vi "Host_HoppingScan(XZ_TargetMultiLayerImage).vi"() -> ()   [LabVIEW 2014]
uses:
  <vilib>/userdefined/High Color/nirio_resource_hc.ctl
  <vilib>/Instr/_visa.llb/VISA Configure Serial Port (Instr).vi
  <vilib>/FPGAPlugInAG/PCIe-7851R/niLvFpga_Open_PCIe-7851R.vi
  <vilib>/rvi/interface/common/dynamic/niFpgaDynamicAddResources.vi
  <vilib>/Utility/error.llb/Error Cluster From Error Code.vi
  <vilib>/rvi/errors/niLvFpgaAdjustHostInterfaceError.vi
  <vilib>/FPGAPlugInAG/Dynamic/niLvFpga_Close_Dynamic.vi
  <vilib>/rvi/interface/nirviOpenFPGA/nirviOpenFPGA.xnode
  FPGA Bitfiles/XZFPGAWithinHopp_FPGATarget_HoppingStep(Nonl_hC1Fmxzhga8.lvbitx
  <vilib>/rvi/interface/nirviReadWriteControl/nirviReadWriteControl.xnode
  <vilib>/rvi/interface/nirviMethod/nirviMethod.xnode
  <vilib>/rvi/interface/nirviCloseFPGA/nirviCloseFPGA.xnode
  NiFpgaLv.dll
  <vilib>/rvi/interface/Simulation/niFpgaSimulationCallBeginRW.vi
  <vilib>/FPGAPlugInAG/Dynamic/niLvFpga_ReadFifo_Dynamic.vi
  <vilib>/rvi/errors/niLvFpgaMergeErrorWithErrorCode.vi
  <vilib>/FPGAPlugInAG/Dynamic/niLvFpga_StopFifo_Dynamic.vi
panel:
  out "RTPlot":i32(graph)
  in  "ScanLayerNum":u32
  in  "LowPassFilter":i32
  out "XGetNum":u32
  in  "BottomSleep us":i32
  in  "UpperSleep us":i32
  out "SecElapsed s":dbl
  in  "UseCompensation":bool
  in  "Compensation / line":i32
  in  "RelativeWithdraw index":i32
  out "YPresPos":i32
  out "XBuffer":u32
  out "LinePlot":i16[](graph)
  in  "stop":bool
  in  "ZOffset index":i32
  out "YPos?":dbl
  in  "YNum":i16
  in  "XNum":i16
  in  "YStepLen um":dbl format="%#_13g"
  in  "XStepMultiplier / 0.5nm":i16
  in  "XInitPos um":dbl format="%#_13g"
  in  "YInitPos um":dbl format="%#_13g"
  in  "PIXZ":T1
  out "ERR?":string
  in  "PIYDigital":refnum<visa-resource-name>
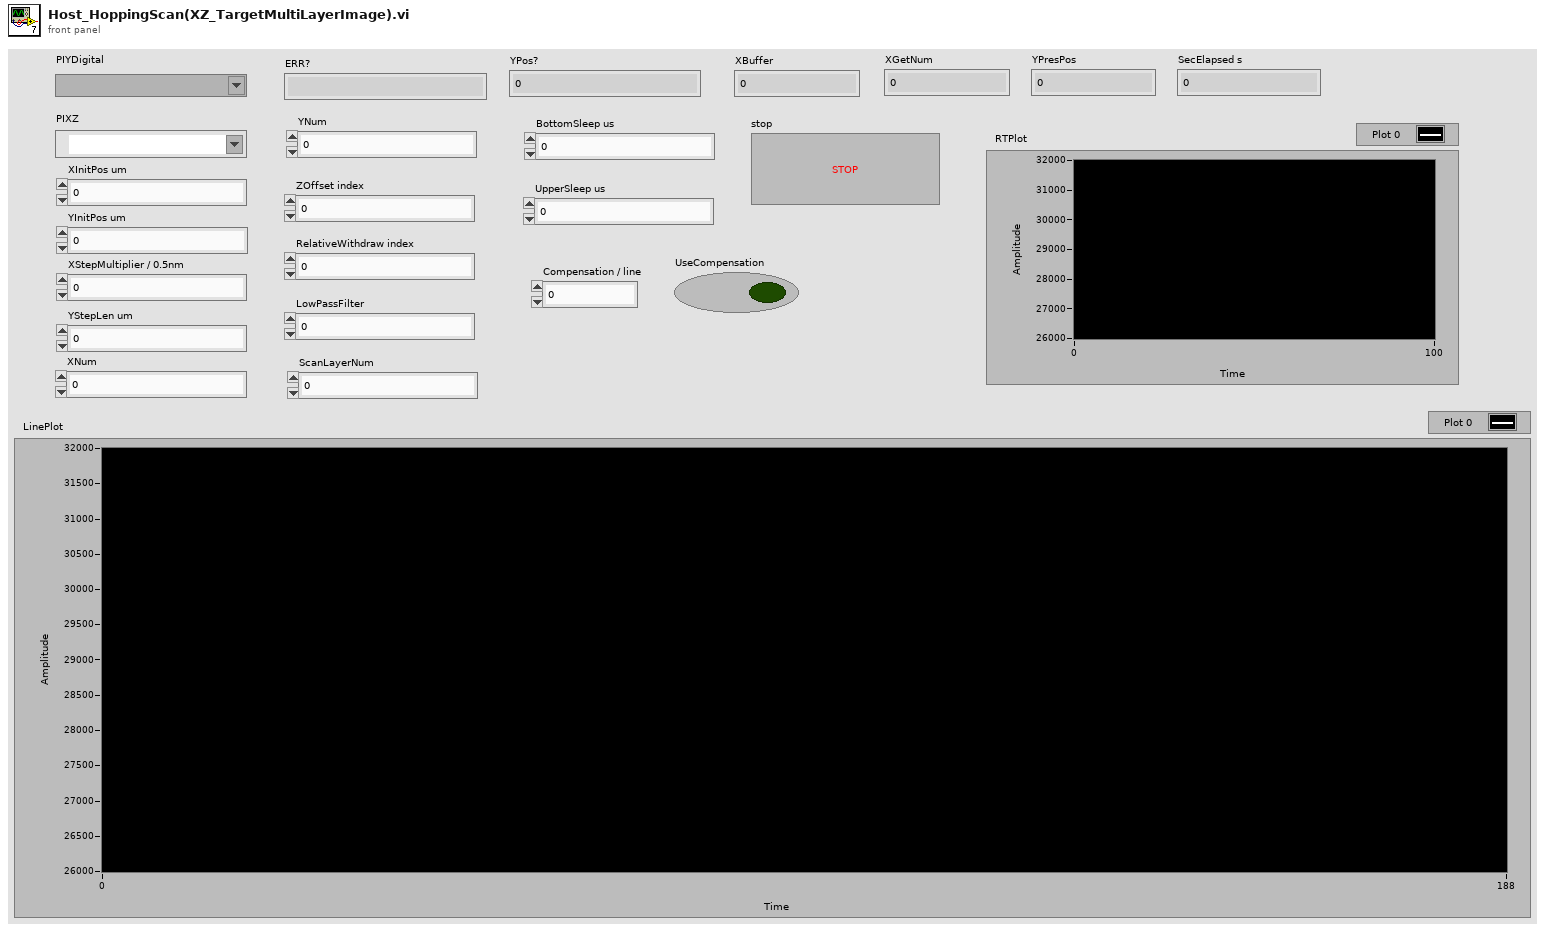
[diagram p1: front panel]
types:
  T1 = typedef "nirio_resource_hc.ctl" = tag
  T2 = enum16{"open", "replace", "create", "open or create", "replace or create", "replace or create with confirmation"}
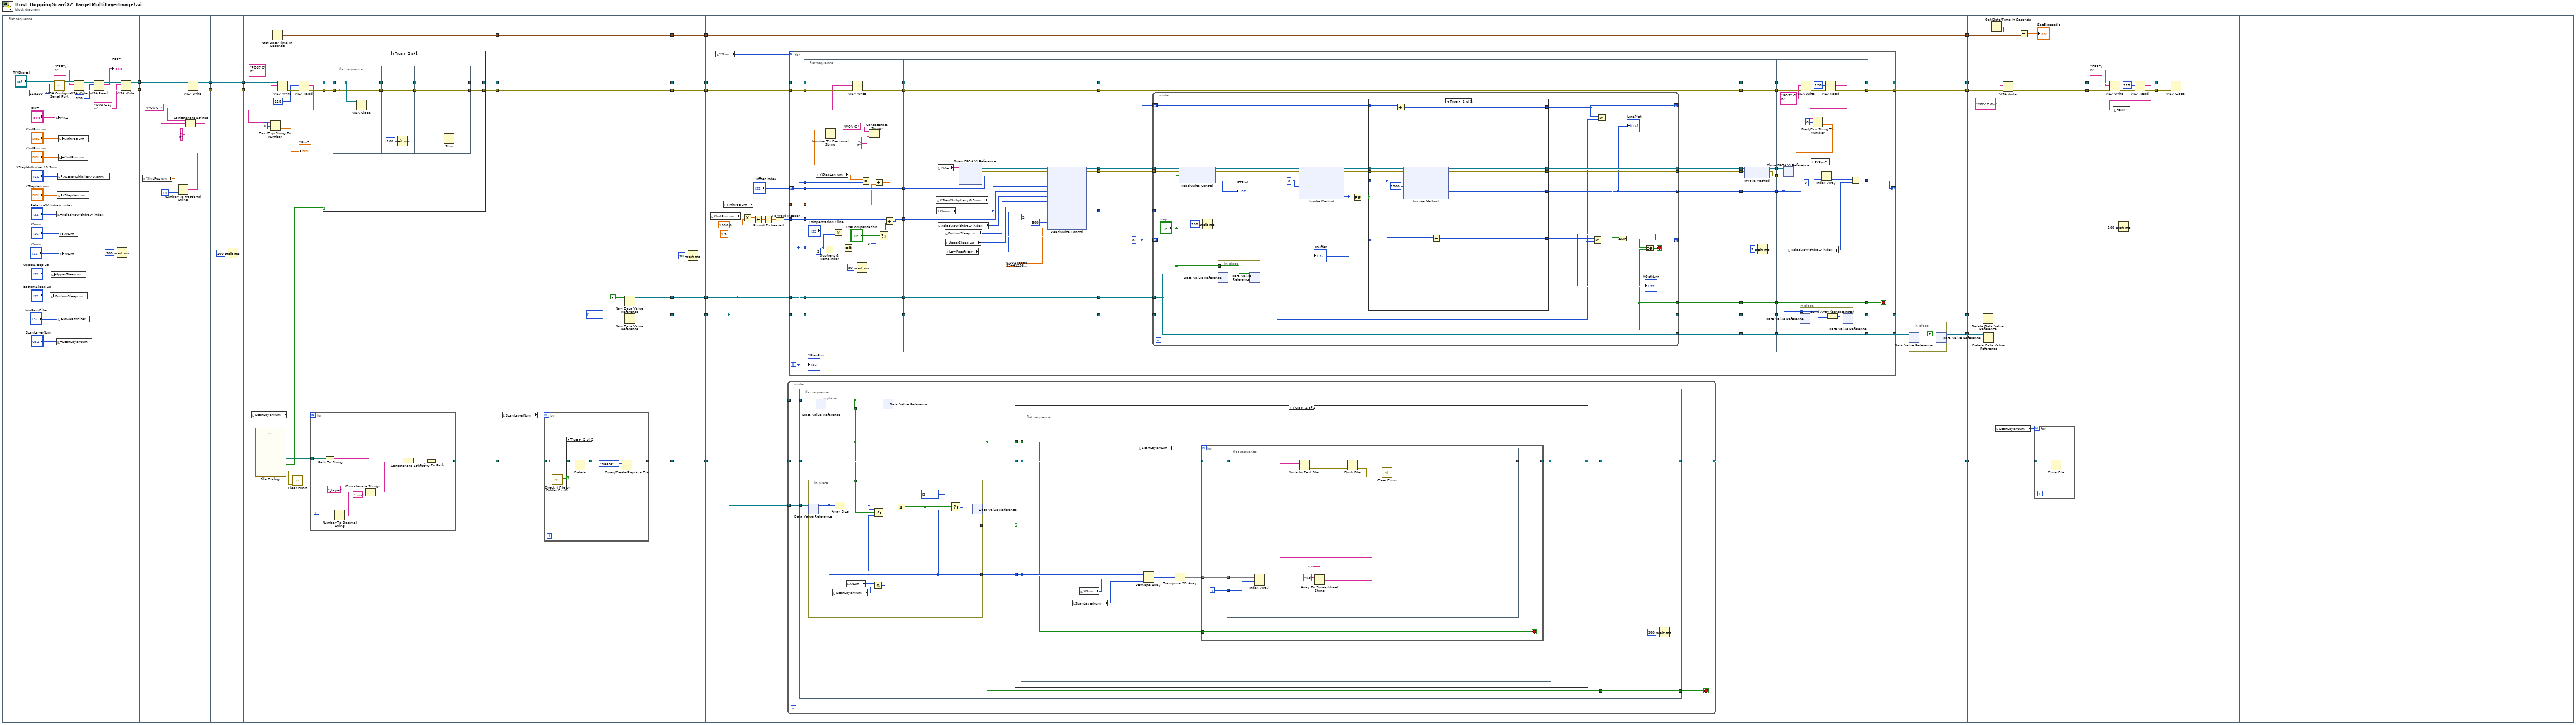
[diagram p0: block diagram]
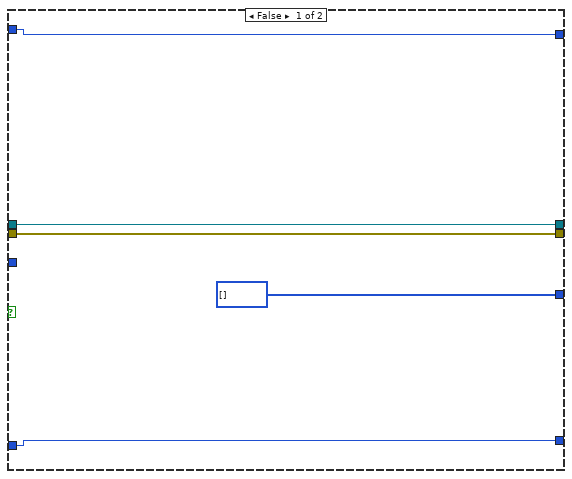
[diagram p5: hidden frame]
diagram:
  n1 = flat-sequence {
    tunnel: [w39] -> w32
    tunnel: [w38] -> w31
    tunnel: w32 -> [w69]
    tunnel: w31 -> [w68]
    tunnel: [w64] -> w30
    tunnel: [w63] -> w29
    tunnel: w30 -> [w71]
    tunnel: w29 -> [w70]
    tunnel: [w71] -> w28
    tunnel: [w70] -> w27
    tunnel: w28 -> [w91]
    tunnel: w27 -> [w90]
    tunnel: [w78] -> w16
    tunnel: [w77] -> w14
    tunnel: [w82] -> w12
    tunnel: [w73] -> w10
    tunnel: w16 -> [w127]
    tunnel: [w127] -> w15
    tunnel: w14 -> [w126]
    tunnel: [w126] -> w13
    tunnel: w12 -> [w125]
    tunnel: [w125] -> w11
    tunnel: w10 -> [w123]
    tunnel: [w122] -> w8
    tunnel: [w120] -> w6
    tunnel: [w118] -> w4
    tunnel: w15 -> [w141]
    tunnel: w13 -> [w140]
    tunnel: [w141] -> w26
    tunnel: [w140] -> w25
    tunnel: [w139] -> w18
    tunnel: w11 -> [w139]
    tunnel: [w138] -> w9
    tunnel: w8 -> [w138]
    tunnel: [w137] -> w7
    tunnel: w6 -> [w137]
    tunnel: [w136] -> w5
    tunnel: w4 -> [w136]
    tunnel: w26 -> [w163]
    tunnel: w25 -> [w162]
    tunnel: [w154] -> w24
    tunnel: [w153] -> w23
    tunnel: w18 -> [w150]
    tunnel: [w150] -> w17
    tunnel: w9 -> [w149]
    tunnel: w7 -> [w148]
    tunnel: w5 -> [w147]
    tunnel: [w145] -> w3
    tunnel: [w144] -> w2
    tunnel: [w143] -> w1
    tunnel: w24 -> [w418]
    tunnel: w23 -> [w417]
    tunnel: [w415] -> w22
    tunnel: [w414] -> w21
    tunnel: w17 -> [w413]
    tunnel: w3 -> [w410]
    tunnel: w2 -> [w408]
    tunnel: w1 -> [w407]
    tunnel: w22 -> [w429]
    tunnel: w21 -> [w428]
    tunnel: [w423] -> w20
    tunnel: [w422] -> w19
    tunnel: w20 -> [w431]
    tunnel: w19 -> [w430]
    frame #0 {
      n2 = local write "BottomSleep us"("BottomSleep us") -> ()
      n3 = local write "UpperSleep us"("UpperSleep us") -> ()
      n4 = call-poly "VISA Configure Serial Port"("VISA resource name"="PIYDigital", "baud rate (9600)"=u32 115200) -> ("VISA resource name out"=w57:refnum<visa-resource-name>, "error out"=w56:errorcluster)  [unwired: 12 in]
      n5 = local write "PIXZ"("PIXZ") -> ()
      n6 = local write "RelativeWithdraw index"("RelativeWithdraw index") -> ()
      n7 = local write "ScanLayerNum"("ScanLayerNum") -> ()
      n8 = local write "YStepLen um"("YStepLen um") -> ()
      n9 = local write "LowPassFilter"("LowPassFilter") -> ()
      n10 = local write "XStepMultiplier / 0.5nm"("XStepMultiplier / 0.5nm") -> ()
      n11 = local write "YInitPos um"("YInitPos um") -> ()
      n12 = local write "XInitPos um"("XInitPos um") -> ()
      n13 = local write "XNum"("XNum") -> ()
      n14 = local write "YNum"("YNum") -> ()
      n15 = VISA Write(VISA resource name=w57, write buffer="ERR?\n", error in (no error)=w56) -> (VISA resource name out=w54:refnum<visa-resource-name>, error out=w53:errorcluster)  [unwired: 1 out]
      n16 = VISA Read(VISA resource name=w54, byte count=u32 128, error in (no error)=w53) -> (VISA resource name out=w41:refnum<visa-resource-name>, read buffer=→"ERR?":string, error out=w40:errorcluster)  [unwired: 1 out]
      n17 = Wait (ms)(milliseconds to wait=u32 500) -> ()  [unwired: 1 out]
      n18 = VISA Write(VISA resource name=w41, write buffer="SVO C 1\n", error in (no error)=w40) -> (VISA resource name out=w39:refnum<visa-resource-name>, error out=w38:errorcluster)  [unwired: 1 out]
    }
    frame #1 {
      n19 = local read "YInitPos um"() -> (w62:dbl)
      n20 = Number To Fractional String(number=w62, precision (6)=i16 10) -> (F-format string=w60:string)  [unwired: 2 in]
      n21 = Concatenate Strings("MOV C  " ("write buffer"), w60, "\n" ("string")) -> (w65:string)
      n22 = VISA Write(VISA resource name=w69, write buffer=w65, error in (no error)=w68) -> (VISA resource name out=w64:refnum<visa-resource-name>, error out=w63:errorcluster)  [unwired: 1 out]
    }
    frame #2 {
      n23 = Wait (ms)(milliseconds to wait=u32 200) -> ()  [unwired: 1 out]
    }
    frame #3 {
      n24 = local read "ScanLayerNum"() -> (w75:u32)
      n25 = call "File Dialog"() -> ("selected path"=w74:path, "cancelled"=w76:bool, "error out"=w81:errorcluster)  [unwired: 12 in, 1 out]
      n26 = Get Date/Time In Seconds() -> (seconds since 1Jan1904=w82:timestamp)
      n27 = VISA Write(VISA resource name=w91, write buffer="POS? C\n", error in (no error)=w90) -> (VISA resource name out=w88:refnum<visa-resource-name>, error out=w87:errorcluster)  [unwired: 1 out]
      n28 = call <vilib>:"Clear Errors.vi"("error in (no error)"=w81) -> ()  [unwired: 5 in, 2 out]
      n29 = VISA Read(VISA resource name=w88, byte count=u32 128, error in (no error)=w87) -> (VISA resource name out=w80:refnum<visa-resource-name>, read buffer=w85:string, error out=w79:errorcluster)  [unwired: 1 out]
      n30 = Fract/Exp String To Number(string=w85, offset=0) -> (number=→"YPos?":dbl)  [unwired: 2 in, 1 out]
      n31 = for {
        N: w75 -> [_]
        tunnel: w74 -> [w96]
        tunnel: [w92] -> w73 mode=indexing
        i -> [w99]
        n32 = Path To String(path=w96) -> (string=w95:string)
        n33 = Number To Decimal String(number=w99) -> (decimal integer string=w98:string)  [unwired: 1 in]
        n34 = Concatenate Strings("_layer" ("string"), w98, ".csv" ("string")) -> (w94:string)
        n35 = Concatenate Strings(w95, w94) -> (w93:string)
        n36 = String To Path(string=w93) -> (path=w92:path)
      }
      n37 = case shown="True" w76 {
        tunnel: w80 -> [w102 w110]
        tunnel: w79 -> [w101 w109]
        tunnel: [w102 w106] -> w78
        tunnel: [w101 w103] -> w77
        frame False {
        }
        frame True {
          n38 = flat-sequence {
            tunnel: w110 -> [w112]
            tunnel: w109 -> [w111]
            tunnel: [w112] -> w107
            tunnel: [w111] -> w104
            tunnel: [w115] -> w108
            tunnel: w107 -> [w115]
            tunnel: [w114] -> w105
            tunnel: w104 -> [w114]
            tunnel: [w117] -> w106
            tunnel: w108 -> [w117]
            tunnel: [w116] -> w103
            tunnel: w105 -> [w116]
            frame #0 {
              n39 = VISA Close(VISA resource name=w112, error in (no error)=w111) -> ()  [unwired: 1 out]
            }
            frame #1 {
              n40 = Wait (ms)(milliseconds to wait=u32 200) -> ()  [unwired: 1 out]
            }
            frame #2 {
              n41 = Stop() -> ()  [unwired: 1 in]
            }
          }
        }
      }
    }
    frame #4 {
      n42 = local read "ScanLayerNum"() -> (w124:u32)
      n43 = for {
        N: w124 -> [_]
        tunnel: w123 -> [w131] mode=indexing
        tunnel: [w128] -> w122 mode=indexing
        n44 = call <vilib>:"Check if File or Folder Exists.vi"("path"=w131) -> ("file or folder exists?"=w132:bool)  [unwired: 8 in, 2 out]
        n45 = case shown="True" w132 {
          tunnel: w131 -> [w133 w135]
          tunnel: [w133 w134] -> w130
          frame False {
          }
          frame True {
            n46 = Delete(path (use dialog)=w135) -> (deleted path=w134:path)  [unwired: 4 in, 2 out]
          }
        }
        n47 = Open/Create/Replace File(file path (use dialog)=w130, operation (0:open)=T2."create") -> (refnum out=w128:refnum<file>)  [unwired: 4 in, 2 out]
      }
      n48 = New Data Value Reference(data value=FALSE) -> (data value reference=w120:refnum<data-value>)  [unwired: 1 in, 1 out]
      n49 = New Data Value Reference(data value=i32[] []) -> (data value reference=w118:refnum<data-value>)  [unwired: 1 in, 1 out]
    }
    frame #5 {
      n50 = Wait (ms)(milliseconds to wait=u32 50) -> ()  [unwired: 1 out]
    }
    frame #6 {
      n51 = local read "XInitPos um"() -> (w156:dbl)
      n52 = local read "YNum"() -> (w164:i16)
      n53 = local read "YInitPos um"() -> (w151:dbl)
      n54 = Multiply(x=w156, y=1000.0) -> (x*y=w158:dbl)
      n55 = Divide(x=w158, y=1.5) -> (x/y=w160:dbl)
      n56 = Round To Nearest(number=w160) -> (nearest integer value=w161:dbl)
      n57 = To Word Integer(number=w161) -> (16bit integer=w155:i16)
      n58 = while {
        tunnel: w149 -> [w172]
        tunnel: w148 -> [w171]
        tunnel: w147 -> [w170]
        tunnel: [w168] -> w145
        stop <- w166 stop-if-true
        n59 = flat-sequence {
          tunnel: w170 -> [w179]
          tunnel: w171 -> [w178]
          tunnel: w172 -> [w176]
          tunnel: [w175] -> w169
          tunnel: [w174] -> w167
          tunnel: [w222] -> w168
          tunnel: w169 -> [w222]
          tunnel: [w221] -> w166
          tunnel: w167 -> [w221]
          frame #0 {
            n60 = in-place {
              in-place-border: [w210] -> w174
              n61 = in-place-dvr #1(w178) -> (w210:bool)  [unwired: 1 out]
              n62 = in-place-dvr #1(w210) -> ()  [unwired: 2 out]
            }
            n63 = in-place {
              in-place-border: [w218] -> w177
              in-place-border: w174 -> [w220]
              in-place-border: [w211] -> w173
              n64 = in-place-dvr #2(w179) -> (w218:i32[])  [unwired: 1 out]
              n65 = local read "ScanLayerNum"() -> (w213:u32)
              n66 = Array Size(array=w218) -> (size(s)=w219:i32)
              n67 = local read "XNum"() -> (w214:i16)
              n68 = Multiply(x=w214, y=w213) -> (x*y=w212:u32)
              n69 = Select(t=w219, s=w220, f=w212) -> (s? t:f=w215:u32)
              n70 = Greater Or Equal?(x=w219, y=w215) -> (x >= y?=w211:bool)
              n71 = Select(t=i32[] [], s=w211, f=w218) -> (s? t:f=w216:i32[])
              n72 = in-place-dvr #2(w216) -> ()  [unwired: 2 out]
            }
            n73 = case shown="True" w173 {
              tunnel: w177 -> [_ w183]
              tunnel: w176 -> [w180 w184]
              tunnel: w174 -> [_ w182]
              tunnel: [w180 w181] -> w175
              frame False {
              }
              frame True {
                n74 = flat-sequence {
                  tunnel: w183 -> [w191]
                  tunnel: w184 -> [w192]
                  tunnel: [w190] -> w181
                  tunnel: w182 -> [w189]
                  frame #0 {
                    n75 = local read "ScanLayerNum"() -> (w187:u32)
                    n76 = local read "XNum"() -> (w188:i16)
                    n77 = local read "ScanLayerNum"() -> (w193:u32)
                    n78 = Reshape Array(w191, w188, w187) -> (w186:i32[][])
                    n79 = Transpose 2D Array(2D array=w186) -> (transposed array=w185:i32[][])
                    n80 = for {
                      N: w193 -> [_]
                      tunnel: w192 -> [w198] mode=indexing
                      tunnel: w185 -> [w197]
                      tunnel: [w195] -> w190 mode=indexing
                      tunnel: w189 -> [w194]
                      i -> [w196]
                      stop <- w194 stop-if-true
                      n81 = flat-sequence {
                        tunnel: w198 -> [w205]
                        tunnel: w197 -> [w209]
                        tunnel: w196 -> [w199]
                        tunnel: [w202] -> w195
                        frame #0 {
                          n82 = Index Array(array=w209, index (row)=w199) -> (element=w208:i32[])  [unwired: 1 in]
                          n83 = Array To Spreadsheet String(delimiter (Tab)=",", array=w208, 3:"%d" ("format string")) -> (spreadsheet string=w200:string)
                          n84 = Write to Text File(file (use dialog)=w205, text=w200) -> (refnum out=w204:refnum<file>, error out=w203:errorcluster)  [unwired: 2 in, 1 out]
                          n85 = Flush File(refnum=w204, error in=w203) -> (refnum out=w202:refnum<file>, error out=w201:errorcluster)
                          n86 = call <vilib>:"Clear Errors.vi"("error in (no error)"=w201) -> ()  [unwired: 5 in, 2 out]
                        }
                      }
                    }
                  }
                }
              }
            }
          }
          frame #1 {
            n87 = Wait (ms)(milliseconds to wait=u32 300) -> ()  [unwired: 1 out]
          }
        }
      }
      n88 = for {
        N: w164 -> [_]
        tunnel: w163 -> [w266]
        tunnel: w162 -> [w265]
        tunnel: w155 -> [w259]
        tunnel: [w251] -> w154
        tunnel: [w250] -> w153
        shift-right: [w236] -> _
        shift-left: "ZOffset index" -> [w242]
        tunnel: w151 -> [w238]
        tunnel: w148 -> [w235]
        tunnel: w147 -> [w232]
        tunnel: [w227] -> w146
        tunnel: [w224] -> w143
        i -> [w241]
        stop <- w237 stop-if-true
        n89 = flat-sequence {
          tunnel: w266 -> [w292]
          tunnel: w265 -> [w291]
          tunnel: w241 -> [w293]
          tunnel: [w290] -> w264
          tunnel: [w289] -> w263
          tunnel: [w275] -> w260
          tunnel: w259 -> [w276]
          tunnel: [w283] -> w243
          tunnel: w242 -> [w283]
          tunnel: w241 -> [w273]
          tunnel: w238 -> [w278]
          tunnel: w235 -> [w268]
          tunnel: [w268] -> w233
          tunnel: w232 -> [w267]
          tunnel: [w267] -> w230
          tunnel: [w310] -> w262
          tunnel: [w309] -> w261
          tunnel: [w306] -> w258
          tunnel: [w305] -> w257
          tunnel: [w300] -> w254
          tunnel: w243 -> [w304]
          tunnel: w260 -> [w307]
          tunnel: w263 -> [w309]
          tunnel: w264 -> [w310]
          tunnel: [w295] -> w234
          tunnel: w233 -> [w295]
          tunnel: [w294] -> w231
          tunnel: w230 -> [w294]
          tunnel: w262 -> [w327]
          tunnel: w261 -> [w326]
          tunnel: w258 -> [w320]
          tunnel: w257 -> [w319]
          tunnel: [w327] -> w256
          tunnel: [w326] -> w255
          tunnel: w254 -> [w325]
          tunnel: [w324] -> w253
          tunnel: [w323] -> w252
          tunnel: [w322] -> w247
          tunnel: [w321] -> w244
          tunnel: w234 -> [w317]
          tunnel: w231 -> [w316]
          tunnel: [w315] -> w228
          tunnel: [w314] -> w225
          tunnel: w256 -> [w381]
          tunnel: w255 -> [w380]
          tunnel: w253 -> [w376]
          tunnel: w252 -> [w375]
          tunnel: [w381] -> w249
          tunnel: [w380] -> w248
          tunnel: w247 -> [w378]
          tunnel: [w378] -> w246
          tunnel: [w377] -> w245
          tunnel: w244 -> [w377]
          tunnel: [w374] -> w240
          tunnel: [w373] -> w239
          tunnel: [w372] -> w229
          tunnel: w228 -> [w372]
          tunnel: [w371] -> w226
          tunnel: w225 -> [w371]
          tunnel: [w400] -> w236
          tunnel: [w402] -> w250
          tunnel: [w403] -> w251
          tunnel: w239 -> [w388]
          tunnel: w240 -> [w389]
          tunnel: w245 -> [w383]
          tunnel: w246 -> [w387]
          tunnel: w248 -> [w398]
          tunnel: w249 -> [w399]
          tunnel: [w387] -> w237
          tunnel: [w385] -> w227
          tunnel: w229 -> [w385]
          tunnel: w226 -> [w384]
          tunnel: [w382] -> w224
          frame #0 {
            n90 = local read "YStepLen um"() -> (w288:dbl)
            n91 = Quotient & Remainder(x=w273, y=2) -> (x-y*floor(x/y)=w281:i32)  [unwired: 1 out]
            n92 = Multiply(x="Compensation / line", y=w273) -> (x*y=w272:i32)
            n93 = Equal To 0?(x=w281) -> ()  [unwired: 1 out]
            n94 = Wait (ms)(milliseconds to wait=u32 50) -> ()  [unwired: 1 out]
            n95 = Multiply(x=w288, y=w293) -> (x*y=w279:dbl)
            n96 = Add(x=w279, y=w278) -> (x+y=w277:dbl)
            n97 = Number To Fractional String(number=w277) -> (F-format string=w287:string)  [unwired: 3 in]
            n98 = Concatenate Strings("MOV C " ("string"), w287, "\n" ("string")) -> (w284:string)
            n99 = VISA Write(VISA resource name=w292, write buffer=w284, error in (no error)=w291) -> (VISA resource name out=w290:refnum<visa-resource-name>, error out=w289:errorcluster)  [unwired: 1 out]
            n100 = Select(t=w272, s="UseCompensation", f=0) -> (s? t:f=w269:i32)
            n101 = Add(x=w276, y=w269) -> (x+y=w275:i32)
          }
          frame #1 {
            n102 = local read "XStepMultiplier / 0.5nm"() -> (w308:i16)
            n103 = local read "XNum"() -> (w300:i16)
            n104 = local read "PIXZ"() -> (w313:T1)
            n105 = local read "RelativeWithdraw index"() -> (w303:i32)
            n106 = local read "BottomSleep us"() -> (w302:i32)
            n107 = local read "UpperSleep us"() -> (w301:i32)
            n108 = local read "LowPassFilter"() -> (w299:i32)
            n109 = xnode "Open FPGA VI Reference"("resource name"=w313) -> ("FPGA VI Reference Out"=w312:refnum<k20>, "error out"=w311:errorcluster)  [unwired: 1 in]
            n110 = xnode "Read/Write Control"("FPGA VI Reference In"=w312, "error in"=w311, "ZOffset"=w304, "XStepIndex"=w308, "XNum"=w300, "XOffset"=w307, "RelativeWithdraw"=w303, "BottomSleep us"=w302, "UpperSleep us"=w301, "LowPassFilter"=w299, "ExtraStepIn"=u32 2, "TimeConstant"=u32 300, "threshold"=sgl 0.0025) -> ("FPGA VI Reference Out"=w306:refnum<k20>, "error out"=w305:errorcluster)
          }
          frame #2 {
            w318 = 0
            n111 = while {
              tunnel: w320 -> [w347]
              tunnel: w319 -> [w346]
              tunnel: w325 -> [w339]
              tunnel: [w350] -> w324
              tunnel: [w349] -> w323
              tunnel: ["stop"] -> w322
              tunnel: [w336] -> w321 mode=concatenating
              shift-right: [w344] -> _
              shift-left: w318 -> [w345]
              shift-right: [w340] -> _
              shift-left: w318 -> [w342]
              tunnel: w317 -> [w332]
              tunnel: w316 -> [w330]
              tunnel: [w332] -> w315
              tunnel: [w330] -> w314
              stop <- w348 stop-if-true
              w343 = u32 0 ("Number of Elements")
              n112 = xnode "Read/Write Control"("FPGA VI Reference In"=w347, "error in"=w346, "stop"="stop") -> ("FPGA VI Reference Out"=w335:refnum<k20>, "error out"=w334:errorcluster, "Waveform Chart"=→"RTPlot":i32)
              n113 = Wait (ms)(milliseconds to wait=u32 100) -> ()  [unwired: 1 out]
              n114 = in-place {
                in-place-border: "stop" -> [w354]
                n115 = in-place-dvr #3(w332) -> ()  [unwired: 2 out]
                n116 = in-place-dvr #3(w354) -> ()  [unwired: 2 out]
              }
              n117 = xnode "Invoke Method"("FPGA VI Reference In"=w335, "error in"=w334, "Number of Elements"=w343, "Timeout (ms)"=w343) -> ("FPGA VI Reference Out"=w352:refnum<k20>, "error out"=w351:errorcluster, "Elements Remaining"=w329:u32)  [unwired: 1 out]
              "XBuffer" <- w329
              n118 = Not Equal To 0?(x=w329) -> (x != 0?=w328:bool)
              n119 = case shown="True" w328 {
                tunnel: w352 -> [w358 w363]
                tunnel: w351 -> [w357 w362]
                tunnel: [w358 w370] -> w350
                tunnel: [w357 w369] -> w349
                tunnel: w345 -> [w355 w368]
                tunnel: [w355 w367] -> w344
                tunnel: w342 -> [w359 w366]
                tunnel: [w359 w365] -> w340
                tunnel: [i16[] [] ("Data") w360] -> w336
                tunnel: w329 -> [_ w361]
                frame False {
                }
                frame True {
                  n120 = Add(x=w366, y=w361) -> (x+y=w365:u32)
                  n121 = xnode "Invoke Method"("FPGA VI Reference In"=w363, "error in"=w362, "Number of Elements"=w361, "Timeout (ms)"=1000) -> ("FPGA VI Reference Out"=w370:refnum<k20>, "error out"=w369:errorcluster, "Data"=w360:i16[])  [unwired: 1 out]
                  n122 = Add(x=w361, y=w368) -> (x+y=w367:u32)
                }
              }
              "XGetNum" <- w344
              "LinePlot" <- w336
              n123 = Greater Or Equal?(x=w344, y=w339) -> (x >= y?=w341:bool)
              n124 = Greater Or Equal?(x=w340, y=w339) -> (x >= y?=w338:bool)
              n125 = And(x=w338, y=w341) -> (x .and. y?=w337:bool)
              n126 = Or(x=w337, y="stop") -> (x .or. y?=w348:bool)
            }
          }
          frame #3 {
            n127 = xnode "Invoke Method"("FPGA VI Reference In"=w376, "error in"=w375) -> ("FPGA VI Reference Out"=w374:refnum<k20>, "error out"=w373:errorcluster)
            n128 = Wait (ms)(milliseconds to wait=u32 5) -> ()  [unwired: 1 out]
          }
          frame #4 {
            n129 = xnode "Close FPGA VI Reference"("FPGA VI Reference In"=w389, "error in"=w388) -> ()  [unwired: 1 out]
            n130 = local read "RelativeWithdraw index"() -> (w390:i32)
            n131 = in-place {
              in-place-border: w383 -> [w404]
              n132 = in-place-dvr #4(w384) -> (w406:i32[])  [unwired: 1 out]
              n133 = Build Array (concatenate)(w406, w404) -> (w405:i32[])
              n134 = in-place-dvr #4(w405) -> (w382:refnum<data-value>)  [unwired: 1 out]
            }
            n135 = VISA Write(VISA resource name=w399, write buffer="POS? C\n", error in (no error)=w398) -> (VISA resource name out=w397:refnum<visa-resource-name>, error out=w396:errorcluster)  [unwired: 1 out]
            n136 = Index Array(array=w383, index=0) -> (element=w391:i16)
            n137 = VISA Read(VISA resource name=w397, byte count=u32 128, error in (no error)=w396) -> (VISA resource name out=w403:refnum<visa-resource-name>, read buffer=w393:string, error out=w402:errorcluster)  [unwired: 1 out]
            n138 = Fract/Exp String To Number(string=w393, offset=0) -> (number=w401:dbl)  [unwired: 2 in, 1 out]
            n139 = local write "YPos?"(w401) -> ()
            n140 = Subtract(x=w391, y=w390) -> (x-y=w400:i32)
          }
        }
        "YPresPos" <- w241
      }
      n141 = in-place {
        n142 = in-place-dvr #5(w146) -> ()  [unwired: 2 out]
        n143 = in-place-dvr #5(TRUE ("data value")) -> (w144:refnum<data-value>)  [unwired: 1 out]
      }
    }
    frame #7 {
      n144 = Delete Data Value Reference(data value reference=w407) -> ()  [unwired: 1 in, 2 out]
      n145 = Delete Data Value Reference(data value reference=w408) -> ()  [unwired: 1 in, 2 out]
      n146 = Get Date/Time In Seconds() -> (seconds since 1Jan1904=w412:timestamp)
      n147 = local read "ScanLayerNum"() -> (w409:u32)
      n148 = VISA Write(VISA resource name=w418, write buffer="MOV C 0\n", error in (no error)=w417) -> (VISA resource name out=w415:refnum<visa-resource-name>, error out=w414:errorcluster)  [unwired: 1 out]
      n149 = Subtract(x=w412, y=w413) -> (x-y=→"SecElapsed s":dbl)
      n150 = for {
        N: w409 -> [_]
        tunnel: w410 -> [w419] mode=indexing
        n151 = Close File(refnum=w419) -> ()  [unwired: 1 in, 2 out]
      }
    }
    frame #8 {
      n152 = VISA Write(VISA resource name=w429, write buffer="ERR?\n", error in (no error)=w428) -> (VISA resource name out=w426:refnum<visa-resource-name>, error out=w425:errorcluster)  [unwired: 1 out]
      n153 = Wait (ms)(milliseconds to wait=u32 100) -> ()  [unwired: 1 out]
      n154 = VISA Read(VISA resource name=w426, byte count=u32 128, error in (no error)=w425) -> (VISA resource name out=w423:refnum<visa-resource-name>, read buffer=w421:string, error out=w422:errorcluster)  [unwired: 1 out]
      n155 = local write "ERR?"(w421) -> ()
    }
    frame #9 {
      n156 = VISA Close(VISA resource name=w431, error in (no error)=w430) -> ()  [unwired: 1 out]
    }
    frame #10 {
    }
  }
